vi "Convert to CPI Module.vi"(8 "error in":errorcluster, 9 "SD Module in":refnum<class "SD Module.lvclass">, 10 "slot ref in":T1 format="%.0x", 11 "module in":refnum<class "Module.lvclass">) -> (0 "error out":errorcluster, 1 "SD Module out":refnum<class "SD Module.lvclass">, 2 "slot ref out":T1 format="%.0x", 3 "module out":refnum<class "Module.lvclass">)   [LabVIEW 2017, in "Scan Engine Scripting.lvlib"]
uses:
  Scan Engine Scripting.lvlib
  Modules.lvlibp/SD Module/SD Module.lvclass
  Modules/Module/Module.lvclass
  <vilib>/NI Veristand/Custom Device API/Custom Device Item Ref.ctl
  Modules/Mode Classes/Counter PWM Input Mode/Counter PWM Input Mode.lvclass
  C:/dev/github.com/debryant/niveristand-scan-engine-ethercat-custom-device/Custom Device Source/Scripting/Modules/Mode Classes/Mode/Mode.lvclass
  Modules/Mode Classes/Controls/counter pwm input channel settings.ctl
  Modules/Channel Classes/PWM Input Channel/Measurement Type.ctl
  12f3473e-bc6f-42be-bdd4-fb515759a5bc.vi
  Modules/Channel Classes/PWM Input Channel/PWM Input Channel.lvclass
  <vilib>/NI Veristand/Custom Device API/Custom Device API.lvlib
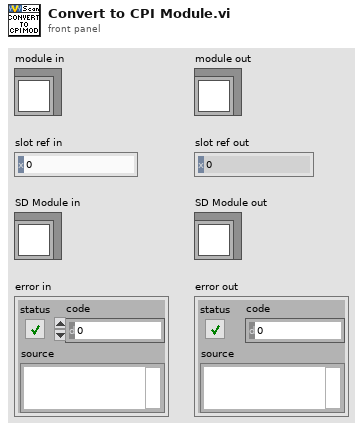
[diagram p1: front panel]
types:
  T1 = typedef "Custom Device API.lvlib/Custom Device Item Ref.ctl" = u64
  T2 = typedef "Scan Engine Scripting.lvlib/counter pwm input channel settings.ctl" = cluster{"name":string, "default value":dbl, "measurement type":T3}
  T3 = typedef "Scan Engine Scripting.lvlib/PWM Input Channel.lvclass/Measurement Type.ctl" = enum16{"High Pulse", "Low Pulse", "Most Recent"}
  T4 = typedef "Modules.lvlibp/SD Module.lvclass/Counter.ctl" = cluster{"Counter Channels":T5[]}
  T5 = typedef "Modules.lvlibp/SD Module.lvclass/Counter Channel.ctl" = cluster{"Measurement Mode":u32, "Count Edges":T6, "Period Measurement":T7, "Pulse Width Measurement":T8, "Frequency Measurement":T9}
  T6 = typedef "Modules.lvlibp/SD Module.lvclass/Count Edges.ctl" = cluster{"Counter Event":u32, "Counter Source":u32, "Counter Direction":u32, "Terminal Count":u32, "Output Mode":u32, "Gate Mode":u32}
  T7 = typedef "Modules.lvlibp/SD Module.lvclass/Period Measurement.ctl" = cluster{"Measurement Edge":u32}
  T8 = typedef "Modules.lvlibp/SD Module.lvclass/Pulse Width Measurement.ctl" = cluster{"Measurement Type":u32}
  T9 = typedef "Modules.lvlibp/SD Module.lvclass/Frequency Measurement.ctl" = cluster{"Measurement Edge":u32, "Measurement Timebase":u32}
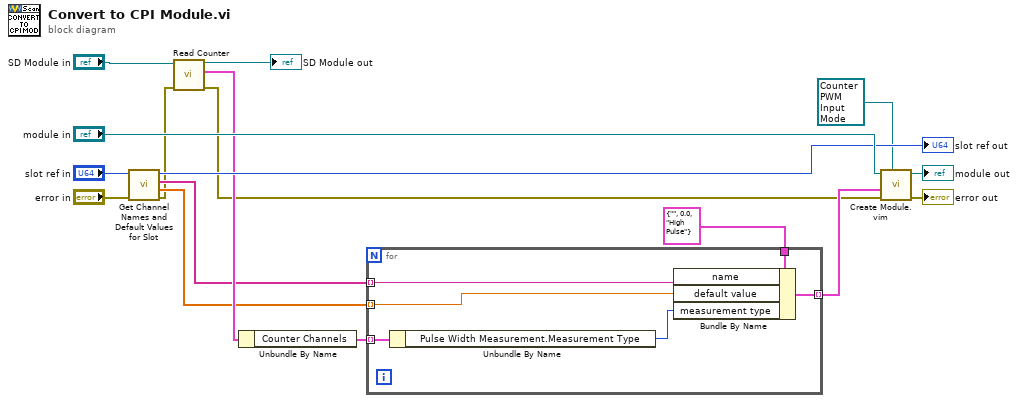
[diagram p0: block diagram]
diagram:
  n1 = call "Get Channel Names and Default Values for Slot.vi"("error in"="error in", "slot ref in"="slot ref in") -> ("error out"=w3:errorcluster, "channel default values"=w6:dbl[], "channel names"=w7:string[], "slot ref out"=→"slot ref out":T1)  [unwired: 6 in]
  n2 = call-dynamic "Read Counter.vi"("error in (no error)"=w3, "SD Module in"="SD Module in") -> ("error out"=w2:errorcluster, "Counter"=w9:T4, "SD Module out"=→"SD Module out":refnum<class "SD Module.lvclass">)  [unwired: 7 in]
  n3 = Unbundle By Name(w9) -> ("Counter Channels"=w8:T5[])
  n4 = for {
    tunnel: w8 -> [w19] mode=indexing
    tunnel: w7 -> [w21] mode=indexing
    tunnel: w6 -> [w20] mode=indexing
    tunnel: T2 {"name"="", "default value"=0.0, "measurement type"=enum."High Pulse"} ("channel settings") -> [w23]
    tunnel: [w22] -> w4 mode=indexing
    n5 = Unbundle By Name(w19) -> ("Pulse Width Measurement.Measurement Type"=w18:u32)
    n6 = Bundle By Name(cluster=w23, "name"=w21, "default value"=w20, "measurement type"=w18) -> (w22:T2)
  }
  n7 = call "Create Module.vim"("mode in"=refnum<class "Counter PWM Input Mode.lvclass"> refnum ("Scan Engine Scripting.lvlib:Counter PWM Input Mode.lvclass"), "error in"=w2, "channel settings"=w4, "module in"="module in") -> ("error out"=→"error out":errorcluster, "module out"=→"module out":refnum<class "Module.lvclass">)  [unwired: 6 in]
